vi "Get Resource.vi"(8 "error in (no error)":errorcluster, 11 "Simulated Waveform in":refnum<class "Simulated Waveform.lvclass">) -> (0 "error out":errorcluster, 2 "Resource":string, 3 "Simulated Waveform out":refnum<class "Simulated Waveform.lvclass">)   [LabVIEW 2020, in "Simulated Waveform.lvlib" / "Simulated Waveform.lvclass"]
uses:
  Simulated Waveform.lvclass
  Simulated Waveform.lvclass/Simulated Waveform.ctl
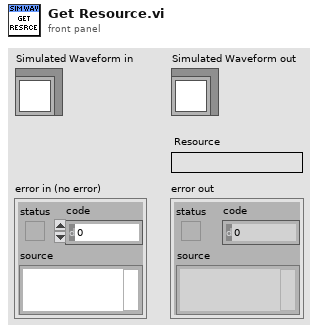
[diagram p1: front panel]
types:
  T1 = typedef "Simulated Waveform.lvlib/Simulated Waveform.lvclass/Ref Data.ctl" = cluster{"Sim Queue Name":string, "Waveform Queue":refnum<queue>, "Noise Factor":dbl}
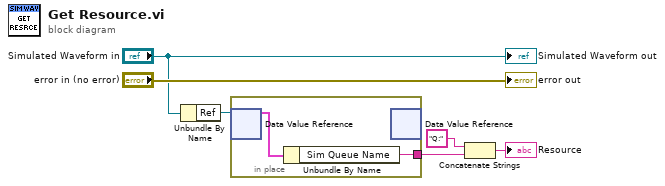
[diagram p0: block diagram]
diagram:
  n1 = Unbundle By Name("Simulated Waveform in") -> ("Ref"=w5:refnum<data-value>)
  n2 = in-place {
    in-place-border: [w7] -> w4
    n3 = in-place-dvr #1(w5) -> (w8:T1)  [unwired: 1 out]
    n4 = Unbundle By Name(w8) -> ("Sim Queue Name"=w7:string)
    n5 = in-place-dvr #1() -> ()  [unwired: 1 in, 2 out]
  }
  n6 = Concatenate Strings("Q:" ("string"), w4) -> (→"Resource":string)
  "error out" <- "error in (no error)"
  "Simulated Waveform out" <- "Simulated Waveform in"
